vi "RunCameraPreview.vi"(8 "error in (no error)":errorcluster, 11 "Point 2":refnum<vi>) -> (0 "error out":errorcluster)   [LabVIEW 2011]
uses:
  Variables/GetPicture.vi
  ccdChipPixels.vi
  lib/System Files/user.lib/atmcd32d.llb/Error Code Enum typedef.ctl
  StopGetPic.vi
panel:
  out "Point":dbl[][](graph)
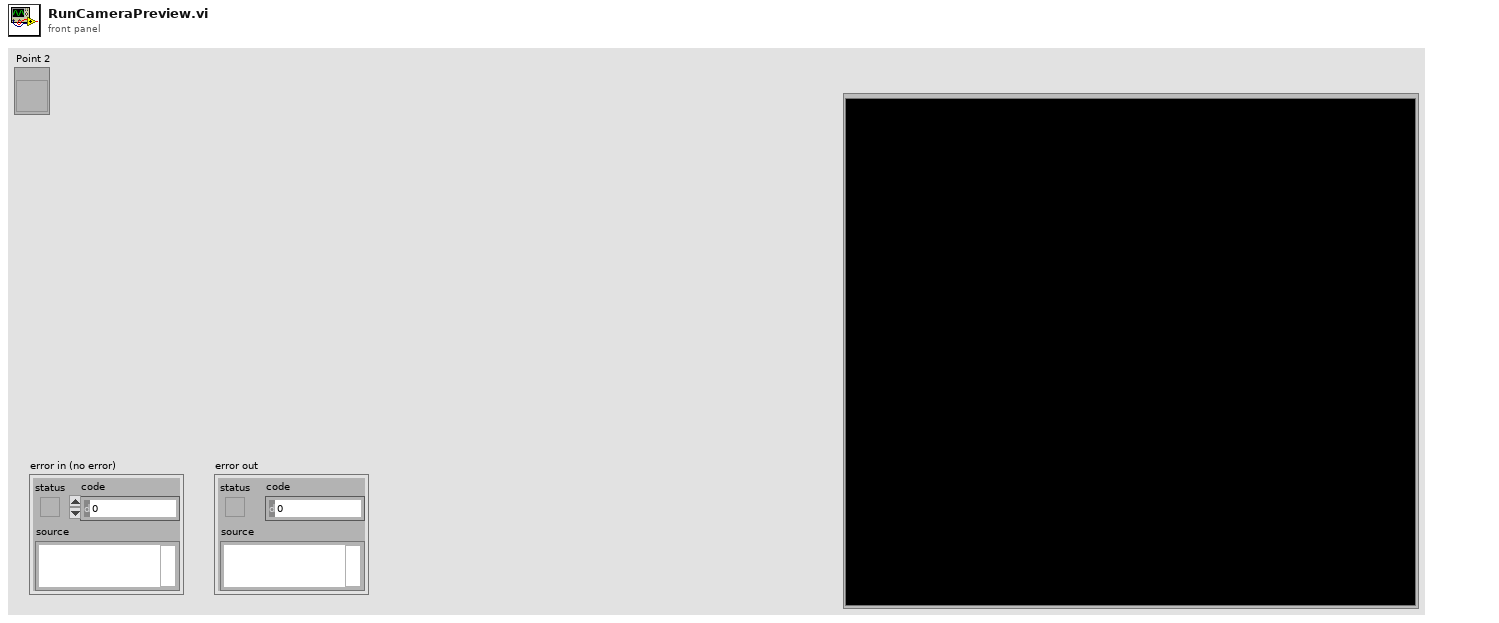
[diagram p1: front panel]
types:
  T1 = typedef "Error Code Enum typedef.ctl" = enum32{"N/A (0)", "DRV_ERROR_CODES", "DRV_SUCCESS", "DRV_VXDNOTINSTALLED", "DRV_ERROR_SCAN", "DRV_ERROR_CHECK_SUM", "DRV_ERROR_FILELOAD", "DRV_UNKNOWN_FUNC", "DRV_ERROR_VXD_INIT", "DRV_ERROR_ADDRESS", "DRV_ERROR_PAGELOCK", "DRV_ERROR_PAGEUNLOCK", "DRV_ERROR_BOARDTEST", "DRV_ERROR_ACK", "DRV_ERROR_UP_FIFO", "DRV_ERROR_PATTERN", "N/A (16)", "DRV_ACQUISITION_ERRORS", "DRV_ACQ_BUFFER", "DRV_ACQ_DOWNFIFO_FULL", "DRV_PROC_UNKONWN_INSTRUCTION", "DRV_ILLEGAL_OP_CODE", "DRV_KINETIC_TIME_NOT_MET", "DRV_ACCUM_TIME_NOT_MET", "DRV_NO_NEW_DATA", "N/A (25)", "DRV_SPOOLERROR", "N/A (27)", "N/A (28)", "N/A (29)", "N/A (30)", "N/A (31)", "N/A (32)", "DRV_TEMPERATURE_CODES", "DRV_TEMPERATURE_OFF", "DRV_TEMPERATURE_NOT_STABILIZED", "DRV_TEMPERATURE_STABILIZED", "DRV_TEMPERATURE_NOT_REACHED", "DRV_TEMPERATURE_OUT_RANGE", "DRV_TEMPERATURE_NOT_SUPPORTED", "DRV_TEMPERATURE_DRIFT", "N/A (41)", "N/A (42)", "N/A (43)", "N/A (44)", "N/A (45)", "N/A (46)", "N/A (47)", "N/A (48)", "DRV_GENERAL_ERRORS", "DRV_INVALID_AUX", "DRV_COF_NOTLOADED", "DRV_FPGAPROG", "DRV_FLEXERROR", "DRV_GPIBERROR", "N/A (55)", "N/A (56)", "N/A (57)", "N/A (58)", "N/A (59)", "N/A (60)", "N/A (61)", "N/A (62)", "N/A (63)", "DRV_DATATYPE", "DRV_DRIVER_ERRORS", "DRV_P1INVALID", "DRV_P2INVALID", "DRV_P3INVALID", "DRV_P4INVALID", "DRV_INIERROR", "DRV_COFERROR", "DRV_ACQUIRING", "DRV_IDLE", "DRV_TEMPCYCLE", "DRV_NOT_INITIALIZED", "DRV_P5INVALID", "DRV_P6INVALID", "DRV_INVALID_MODE", "DRV_INVALID_FILTER", "DRV_I2CERRORS", "DRV_I2CDEVNOTFOUND", "DRV_I2CTIMEOUT", "DRV_P7INVALID", "N/A (84)", "N/A (85)", "N/A (86)", "N/A (87)", "N/A (88)", "N/A (89)", "DRV_IOCERROR", "DRV_VRMVERSIONERROR"}
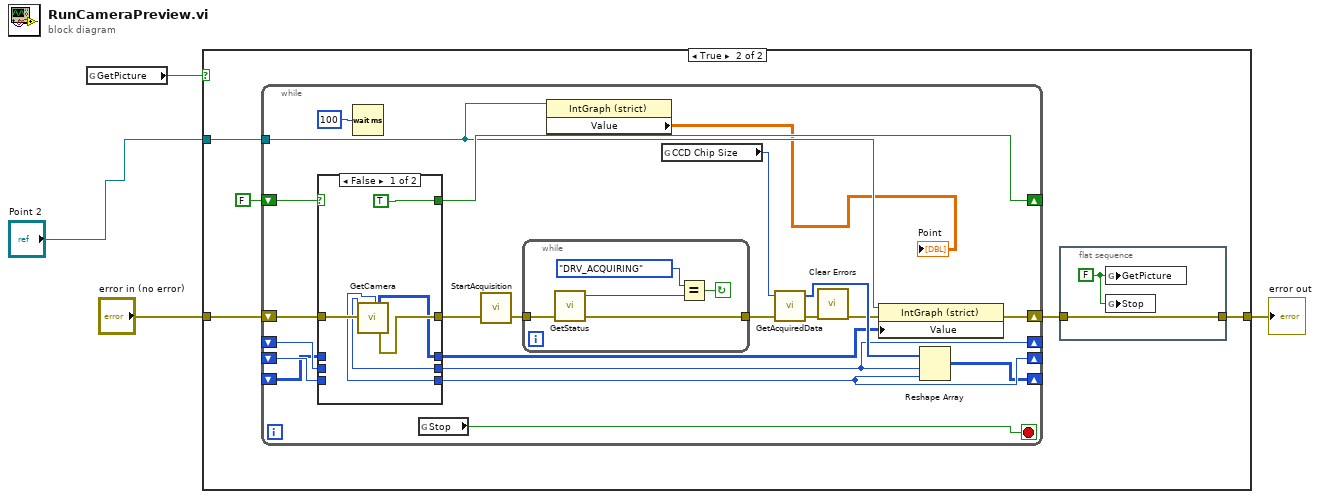
[diagram p0: block diagram]
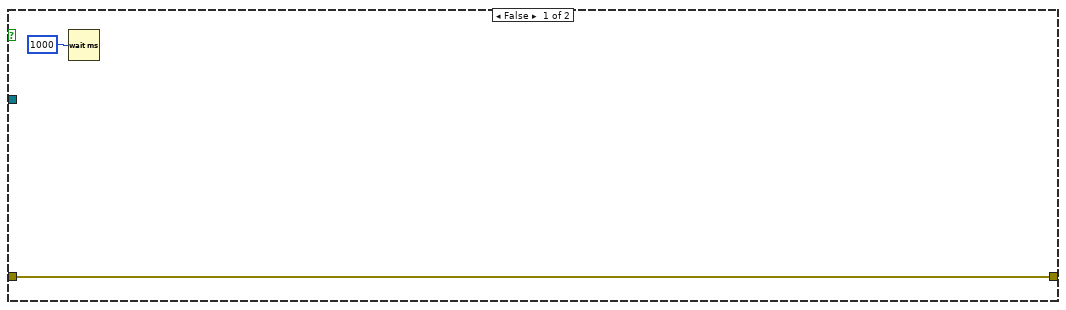
[diagram p2: hidden frame]
diagram:
  n1 = global read "GetPicture.vi" "GetPicture"() -> (w2:bool)
  n2 = case shown="True" w2 {
    tunnel: "error in (no error)" -> [w6 w10]
    tunnel: [w6 w9] -> w4
    tunnel: "Point 2" -> [_ w7]
    frame False {
      n3 = Wait (ms)(milliseconds to wait=u32 1000) -> ()  [unwired: 1 out]
    }
    frame True {
      n4 = while {
        shift-right: [w20] -> w8
        shift-left: w10 -> [w33]
        shift-right: [w27] -> _
        shift-left: FALSE -> [w21]
        shift-right: [w25] -> _
        shift-left: _ -> [w24]
        shift-right: [w26] -> _
        shift-left: _ -> [w23]
        shift-right: [w12] -> _
        shift-left: _ -> [w22]
        tunnel: w7 -> [w14]
        stop <- w18 stop-if-true
        n5 = case shown="False" w21 {
          selector: w21 -> [_ w40]
          tunnel: w33 -> [w39 w44]
          tunnel: [w36 w41] -> w17
          tunnel: [w38 w44] -> w28
          tunnel: [TRUE w40] -> w27
          tunnel: [w35 w43] -> w25
          tunnel: [w34 w42] -> w26
          tunnel: w24 -> [_ w43]
          tunnel: w23 -> [_ w42]
          tunnel: w22 -> [_ w41]
          frame False {
            n6 = call "GetCamera.vi"("error out 2"=w39) -> ("CCD Chip horizontal end"=w35:i32, "CCD Chip Vertical end"=w34:i32, "array"=w36:i32[][], "error out"=w38:errorcluster)  [unwired: 20 in, 3 out]
          }
          frame True {
          }
        }
        n7 = Wait (ms)(milliseconds to wait=u32 100) -> ()  [unwired: 1 out]
        n8 = global read "StopGetPic.vi" "Stop"() -> (w18:bool)
        n9 = call "StartAcquisition.vi"("error in (no error)"=w28) -> ("error out"=w31:errorcluster)  [unwired: 1 in, 1 out]
        n10 = while {
          tunnel: w31 -> [w49]
          tunnel: [w48] -> w30
          stop <- w45 continue-if-true
          n11 = call "GetStatus.vi"("error in (no error)"=w49) -> ("error out"=w48:errorcluster, "status"=w46:T1)  [unwired: 2 in, 1 out]
          n12 = Equal?(x=Error_Code_Enum_typedef."DRV_ACQUIRING" ("status"), y=w46) -> (x = y?=w45:bool)
        }
        n13 = property class="IntGraph (strict)"(reference=w14) -> ("Value"=→"Point":dbl[][])  [unwired: 1 in, 2 out]
        n14 = global read "ccdChipPixels.vi" "CCD Chip Size"() -> (w15:i32)
        n15 = call "GetAcquiredData.vi"("error in (no error)"=w30, "size"=w15) -> ("error out"=w29:errorcluster, "array"=w32:i32[])  [unwired: 1 in, 1 out]
        n16 = call <vilib>:"Clear Errors.vi"("error in (no error)"=w29) -> ("error out"=w16:errorcluster)  [unwired: 6 in]
        n17 = property on="Property Node" class="IntGraph (strict)"(reference=w14, error in=w16, "Value"=w17) -> (error out=w20:errorcluster)  [unwired: 1 out]
        n18 = Reshape Array(w32, w25, w26) -> (w12:i32[][])
      }
      n19 = flat-sequence {
        tunnel: [w51] -> w9
        tunnel: w8 -> [w51]
        frame #0 {
          w50 = FALSE ("GetPicture")
          n20 = global write "GetPicture.vi" "GetPicture"(w50) -> ()
          n21 = global write "StopGetPic.vi" "Stop"(w50) -> ()
        }
      }
    }
  }
  "error out" <- w4
